vi "Lumped element compensation.vi"(6 "Inductance (nH)":dbl, 7 "Capacitance (pF)":dbl, 9 "Subtract stub":bool, 10 "Frequencies (Hz)":dbl[](array[numeric]), 11 "Y/Z Array Out in":cdb[][](array[numeric])) -> (3 "Y/Z Array Out out":cdb[][](array[numeric]))   [LabVIEW 2020]
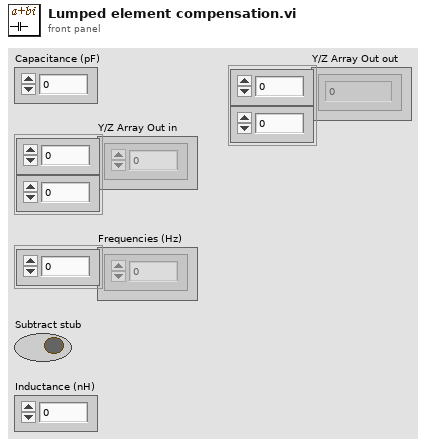
[diagram p1: front panel]
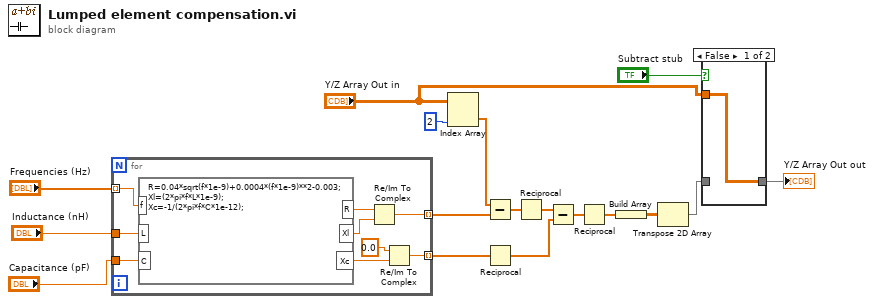
[diagram p0: block diagram]
diagram:
  n1 = for {
    tunnel: "Frequencies (Hz)" -> [w23] mode=indexing
    tunnel: [w24] -> w6 mode=indexing
    tunnel: [w21] -> w11 mode=indexing
    tunnel: "Inductance (nH)" -> [w19]
    tunnel: "Capacitance (pF)" -> [w18]
    n2 = formula code="R=0.04*sqrt(f*1e-9)+0.0004*(f*1e-9)**2-0.003;\nXl=(2*pi*f*L*1e-9);\nXc=-1/(2*pi*f*C*1e-12);"("f"=w23, "L"=w19, "C"=w18) -> ("R"=w26:dbl, "Xl"=w25:dbl, "Xc"=w22:dbl)
    n3 = Re/Im To Complex(1:w25, 2:w26) -> (0:w24:cdb)
    n4 = Re/Im To Complex(1:w22, 2:0.0 ("x")) -> (0:w21:cdb)
  }
  n5 = Index Array(array="Y/Z Array Out in", index (col)=2 ("disabled index (col)")) -> (element=w9:cdb[])  [unwired: 1 in]
  n6 = Subtract(x=w9, y=w6) -> (x-y=w10:cdb[])
  n7 = Reciprocal(x=w11) -> (1/x=w13:cdb[])
  n8 = Reciprocal(x=w10) -> (1/x=w12:cdb[])
  n9 = Subtract(x=w12, y=w13) -> (x-y=w14:cdb[])
  n10 = Reciprocal(x=w14) -> (1/x=w15:cdb[])
  n11 = Build Array(w15) -> (w3:cdb[][])
  n12 = Transpose 2D Array(2D array=w3) -> (transposed array=w7:cdb[][])
  n13 = case shown="False" "Subtract stub" {
    tunnel: [w27 w28] -> w2
    tunnel: "Y/Z Array Out in" -> [w27 _]
    tunnel: w7 -> [_ w28]
    frame False {
    }
    frame True {
    }
  }
  "Y/Z Array Out out" <- w2
